vi "Disarm.vi"(8 "error in (no error)":errorcluster, 9 "Request type":T1=enum."User command", 11 "Ni-Scope Digitizer in":refnum<class "Ni-Scope Digitizer.lvclass">) -> (0 "error out":errorcluster, 2 "Armed":bool, 3 "Ni-Scope Digitizer out":refnum<class "Ni-Scope Digitizer.lvclass">)   [LabVIEW 2021, in "Ni-Scope Digitizer.lvclass"]
uses:
  Ni-Scope Digitizer.lvclass
  Ni-Scope Digitizer.lvclass/Ni-Scope Digitizer.ctl
  Instruments/Pulse Driver/Pulse Driver.lvclass
  LabActor/Controllers/Process Controller/Request type.ctl
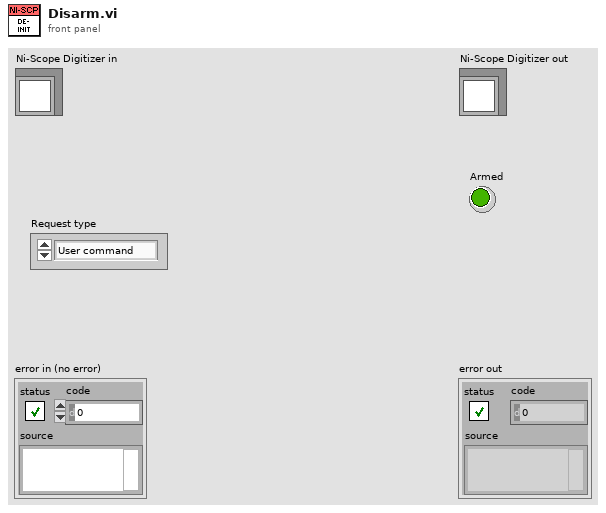
[diagram p1: front panel]
types:
  T1 = typedef "Request type.ctl" = enum16{"Process complete", "User command", "Auto-restart", "Error"}
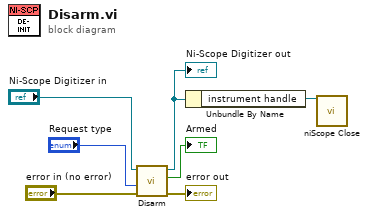
[diagram p0: block diagram]
diagram:
  n1 = call-parent "Disarm.vi"("error in (no error)"="error in (no error)", "Request type"="Request type", "Pulse Driver in"="Ni-Scope Digitizer in") -> ("error out"=→"error out":errorcluster, "Armed"=→"Armed":bool, "Pulse Driver out"=w4:refnum<class "Ni-Scope Digitizer.lvclass">)  [unwired: 6 in]
  "Ni-Scope Digitizer out" <- w4
  n2 = Unbundle By Name(w4) -> ("instrument handle"=w7:refnum<k15>)
  n3 = call <instrlib>:"niScope Close.vi"("instrument handle"=w7) -> ()  [unwired: 14 in, 1 out]
